vi "Read LEMP.vi"(8 "error in (no error)":errorcluster, 11 "FEA_Model in":refnum<class "FEA_Model.lvclass">) -> (0 "error out":errorcluster, 2 "LEMP":T1, 3 "FEA_Model out":refnum<class "FEA_Model.lvclass">)   [LabVIEW 2021, in "FEA_Model.lvclass"]
uses:
  FEA_Model.lvclass
  FEA_Model.lvclass/FEA_Model.ctl
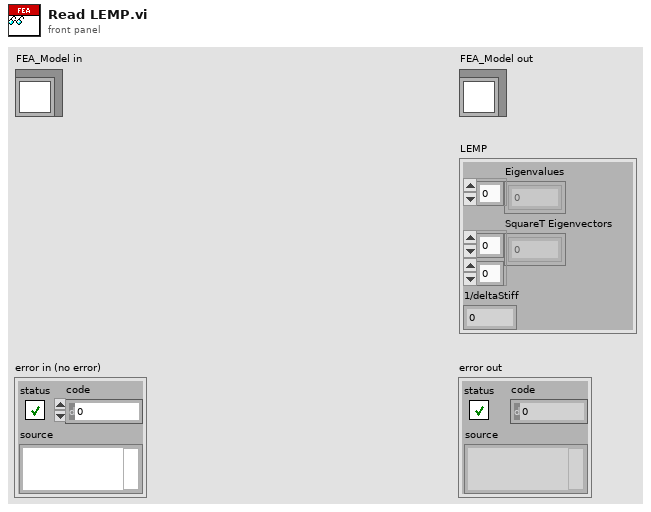
[diagram p1: front panel]
types:
  T1 = cluster{"Eigenvalues":dbl[], "SquareT Eigenvectors":dbl[][], "1/deltaStiff":dbl}
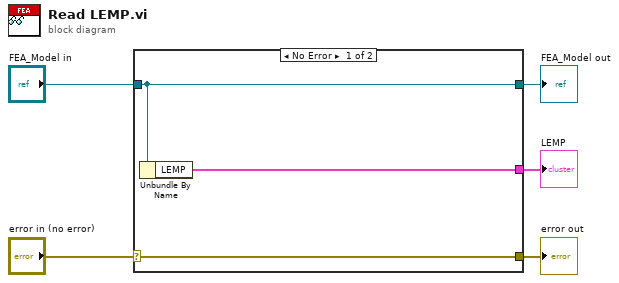
[diagram p0: block diagram]
diagram:
  n1 = case shown="No Error" "error in (no error)" {
    selector: "error in (no error)" -> [w8 w9]
    tunnel: [w8 w9] -> w4
    tunnel: [w7 w10] -> w2
    tunnel: "FEA_Model in" -> [w7 w10]
    tunnel: [w6 _] -> w1
    frame No Error {
      n2 = Unbundle By Name(w7) -> ("LEMP"=w6:T1)
    }
    frame Error {
    }
  }
  "error out" <- w4
  "FEA_Model out" <- w2
  "LEMP" <- w1
